vi "MainIdent RT.vi"() -> ()   [LabVIEW 2019]
doc: "The myRIO Project template acquires acceleration data from the onboard accelerometer and displays the changes of acceleration values in a waveform chart."
uses:
  <vilib>/myRIO/Common/Instrument Driver Framework/myRIO v1.0/Encoder/typedefs/Encoder Signal Mode.ctl
  <vilib>/Platform/TimedLoop/XDataNode/timing_clust.ctl
  <vilib>/Platform/TimedLoop/XDataNode/nitl_modes.ctl
  <vilib>/Platform/TimedLoop/XDataNode/wakeup.ctl
  CD1.ctl
  <vilib>/myRIO/Instrument Drivers/Onboard IO/DIO/typedefs/DIO Reference.ctl
  <vilib>/myRIO/Common/Instrument Driver Framework/Utilities/typedefs/myRIO Generic Hardware Reference.ctl
  <vilib>/myRIO/Common/Instrument Driver Framework/Utilities/typedefs/Hardware Version Enum.ctl
  <vilib>/myRIO/Common/Instrument Driver Framework/Utilities/typedefs/myRIO v1.0 Reference.ctl
  <vilib>/myRIO/Common/Instrument Driver Framework/Utilities/typedefs/Generic FPGA Reference.ctl
  <vilib>/myRIO/Common/Instrument Driver Framework/myRIO v1.0/DIO/typedefs/DIO Channels List.ctl
  <vilib>/myRIO/Common/Instrument Driver Framework/myRIO v1.0/DIO/typedefs/DIO Channels Enum.ctl
  <vilib>/userDefined/High Color/nirio_resource_hc.ctl
  <vilib>/myRIO/Common/Instrument Driver Framework/myRIO v1.0/DIO/vis/myRIO v1.1 Open DIO.vi
  3447d3bf-b8a8-43f1-b6f9-cc57a033e7fd.vi
  468b4709-11a8-4de7-9d16-8f3761c489fc.vi
  a2f579e5-2875-4057-bc92-a0e59aafcda8.vi
  <vilib>/myRIO/Common/Instrument Driver Framework/Utilities/vis/Validate Channels.vi
  <vilib>/myRIO/Common/Instrument Driver Framework/myRIO v1.0/DIO/vis/myRIO v1.0 Reserve DIO.vi
  <vilib>/myRIO/Common/Instrument Driver Framework/myRIO v1.0/UART/vis/myRIO v1.0 Close UART.vi
  <vilib>/myRIO/Common/Instrument Driver Framework/myRIO v1.0/Resource Manager/vis/myRIO v1.0 Reserve Channel List.vi
  <vilib>/myRIO/Common/Instrument Driver Framework/myRIO v1.0/DIO/vis/myRIO v1.0 Build MUX Configuration DIO.vi
  <vilib>/myRIO/Common/Instrument Driver Framework/myRIO v1.0/Resource Manager/vis/myRIO v1.0 Reserve Channel.vi
  <vilib>/myRIO/Common/Instrument Driver Framework/myRIO v1.0/Resource Manager/vis/myRIO v1.0 Unreserve Channel.vi
  <vilib>/myRIO/Common/Instrument Driver Framework/myRIO v1.0/Resource Manager/vis/myRIO v1.0 Create Configuration List.vi
  <vilib>/myRIO/Common/Instrument Driver Framework/myRIO v1.0/Resource Manager/vis/myRIO v1.0 Build Mutex Name.vi
  <vilib>/imath/engines/lvmath2/RunTimeEngine/IndexRead/NIMS V(S).vi
  <instcachedir>/0/NIMS V(S)_0488751826AF41519A22953C041130DC.lvgen/NIMS V(S)_0488751826AF41519A22953C041130DC_000.vi
  <vilib>/imathl/engines/lvmath/Functions/Error Handling/Create Error.vi
  <vilib>/imath/engines/lvmath2/RunTimeEngine/ErrorHandling/NIMS_Create Error From Enums.vi
  <vilib>/imath/engines/lvmath2/RunTimeEngine/RangeToken/NIMS_Range_R3 - Integer.vi
  <instcachedir>/0/NIMS_Range_R3 - Integer_E6E7B420460D4F08A65C42474AF91D7C.lvgen/NIMS_Range_R3 - Integer_E6E7B420460D4F08A65C42474AF91D7C_000.vi
  <vilib>/imath/engines/lvmath2/RunTimeEngine/CommandStatement/MC_CommandStatement_break.vi
  <vilib>/imath/engines/lvmath2/RunTimeEngine/VariableToken/NIMS_VariableToken_CondDefinedDefinedByReplace.vi
  <instcachedir>/0/NIMS_VariableToken_CondDefinedDefinedByReplace_D162CFFC24174562A9FEA619A91E1A56.lvgen/NIMS_VariableToken_CondDefinedDefinedByReplace_D162CFFC24174562A9FEA619A91E1A56_003.vi
  <vilib>/imath/engines/lvmath2/RunTimeEngine/IndexReplace/NIMS V(S)=S.vi
  <instcachedir>/0/NIMS V(S)=S_BD5C8CB81B6E4D99B8C0034EA1BEE55D.lvgen/NIMS V(S)=S_BD5C8CB81B6E4D99B8C0034EA1BEE55D_000.vi
  <vilib>/imath/engines/lvmath2/RunTimeEngine/VariableToken/NIMS_VariableToken_CondDefined.vi
  <instcachedir>/0/NIMS_VariableToken_CondDefined_30C3C94EAC01413DA882E848DEC89944.lvgen/NIMS_VariableToken_CondDefined_30C3C94EAC01413DA882E848DEC89944_004.vi
  <vilib>/imath/engines/lvmath/Functions/Error Handling/MergeErrorsWrapper.vi
  <vilib>/imath/engines/lvmath2/RunTimeEngine/NodeEndStatement/NIMS_NodeEndStatement_Output.vi
  <instcachedir>/0/NIMS_NodeEndStatement_Output_53EC0D466D134D7ABD903AC30B43404B.lvgen/NIMS_NodeEndStatement_Output_53EC0D466D134D7ABD903AC30B43404B_001.vi
  <instcachedir>/0/NIMS_NodeEndStatement_Output_53EC0D466D134D7ABD903AC30B43404B.lvgen/NIMS_NodeEndStatement_Output_53EC0D466D134D7ABD903AC30B43404B_005.vi
  <vilib>/imath/engines/lvmath2/RunTimeEngine/ErrorHandling/NIMS_Finalize Error.vi
  <vilib>/Utility/VariantDataType/GetNumericInfo.vi
  <vilib>/Utility/error.llb/Error Cluster From Error Code.vi
  <vilib>/myRIO/Common/Instrument Driver Framework/myRIO v1.0/myRIO v1.1 Open.vi
  <vilib>/myRIO/Common/Instrument Driver Framework/Utilities/vis/IO Manager.vi
  <vilib>/myRIO/Common/Instrument Driver Framework/Utilities/vis/Configuration Manager.vi
  <vilib>/myRIO/Common/Instrument Driver Framework/myRIO v1.0/Resource Manager/vis/myRIO v1.0 Configure IO.vi
  <vilib>/myRIO/Common/Instrument Driver Framework/myRIO v1.0/myRIO v1.0 Close.vi
  <vilib>/myRIO/Common/Instrument Driver Framework/myRIO v1.0/DIO/vis/myRIO v1.0 Read DIO.vi
  <vilib>/myRIO/Common/Instrument Driver Framework/myRIO v1.0/Encoder/vis/myRIO v1.0 Read Encoder.vi
  <vilib>/myRIO/Common/Instrument Driver Framework/myRIO v1.0/DIO/vis/myRIO v1.0 Write DIO.vi
  <vilib>/myRIO/Common/Instrument Driver Framework/myRIO v1.0/PWM/vis/myRIO v1.0 Write PWM.vi
  <vilib>/myRIO/Common/Instrument Driver Framework/Utilities/vis/FPGA Ref Manager.vi
  <vilib>/myRIO/Common/Instrument Driver Framework/myRIO v1.0/myRIO v1.0 Reset FPGA.vi
  <vilib>/myRIO/Common/Instrument Driver Framework/myRIO v1.0/IRQ/vis/myRIO v1.0 IRQ Info FGV.vi
  <vilib>/myRIO/Common/Instrument Driver Framework/myRIO v1.0/IRQ/vis/myRIO v1.0 Timer IRQ Info FGV.vi
  <vilib>/myRIO/Common/Instrument Driver Framework/myRIO v1.0/IRQ/vis/myRIO v1.0 ISR Agent.vi
  <vilib>/myRIO/Instrument Drivers/Utilities/vis/Reset Index.vi
  <vilib>/myRIO/Common/Instrument Driver Framework/myRIO v1.0/Resource Manager/vis/myRIO v1.0 Block Write Resource Manager.vi
  <vilib>/platform/TimedLoop/XDataNode/XDataNode.xnode
  <vilib>/myRIO/Instrument Drivers/Onboard IO/DIO/vis/myRIO DIO Open.xnode
  <vilib>/Platform/TimedLoop/XDataNode/XDNodeRunTimeDep.lvlib
  <vilib>/myRIO/Instrument Drivers/Onboard IO/Encoder/Encoder.lvlib
  <vilib>/myRIO/Instrument Drivers/Onboard IO/PWM/PWM.lvlib
  <vilib>/myRIO/Instrument Drivers/Onboard IO/DIO/DIO.lvlib
  <vilib>/myRIO/Instrument Drivers/Utilities/Utilities.lvlib
panel:
  out "SetPoint Control 4":dbl
  out "Boolean":bool
  out "SetPoint Control 3":dbl
  out "Pos act":dbl
  out "tt_1":dbl[](array[numeric])
  out "SetPoint Control 2":dbl
  out "Td2":dbl
  out "Ti2":dbl
  out "Kp2":dbl
  out "Td1":dbl
  out "Ti1":dbl
  out "Kp1":dbl
  in  "Wc filtro digital 2":dbl
  in  "Wc filtro digital":dbl
  out "Tiempo de muestreo":dbl
  out "Pulsos 1":i32
  out "Pulsos 2":i32
  out "?":cluster{dbl, dbl}(graph)
  out "?":cluster{dbl, dbl}(graph)
  out "Angulo Motor 1":dbl
  out "Angulo Motor 2":dbl
  out "Velocidad Motor1":dbl caption="rad/s"
  out "Velocidad Motor2":dbl caption="rad/s"
  out "Waveform Chart":dbl(graph)
  in  "error":dbl
  in  "error 2":dbl
  out "Numeric":dbl
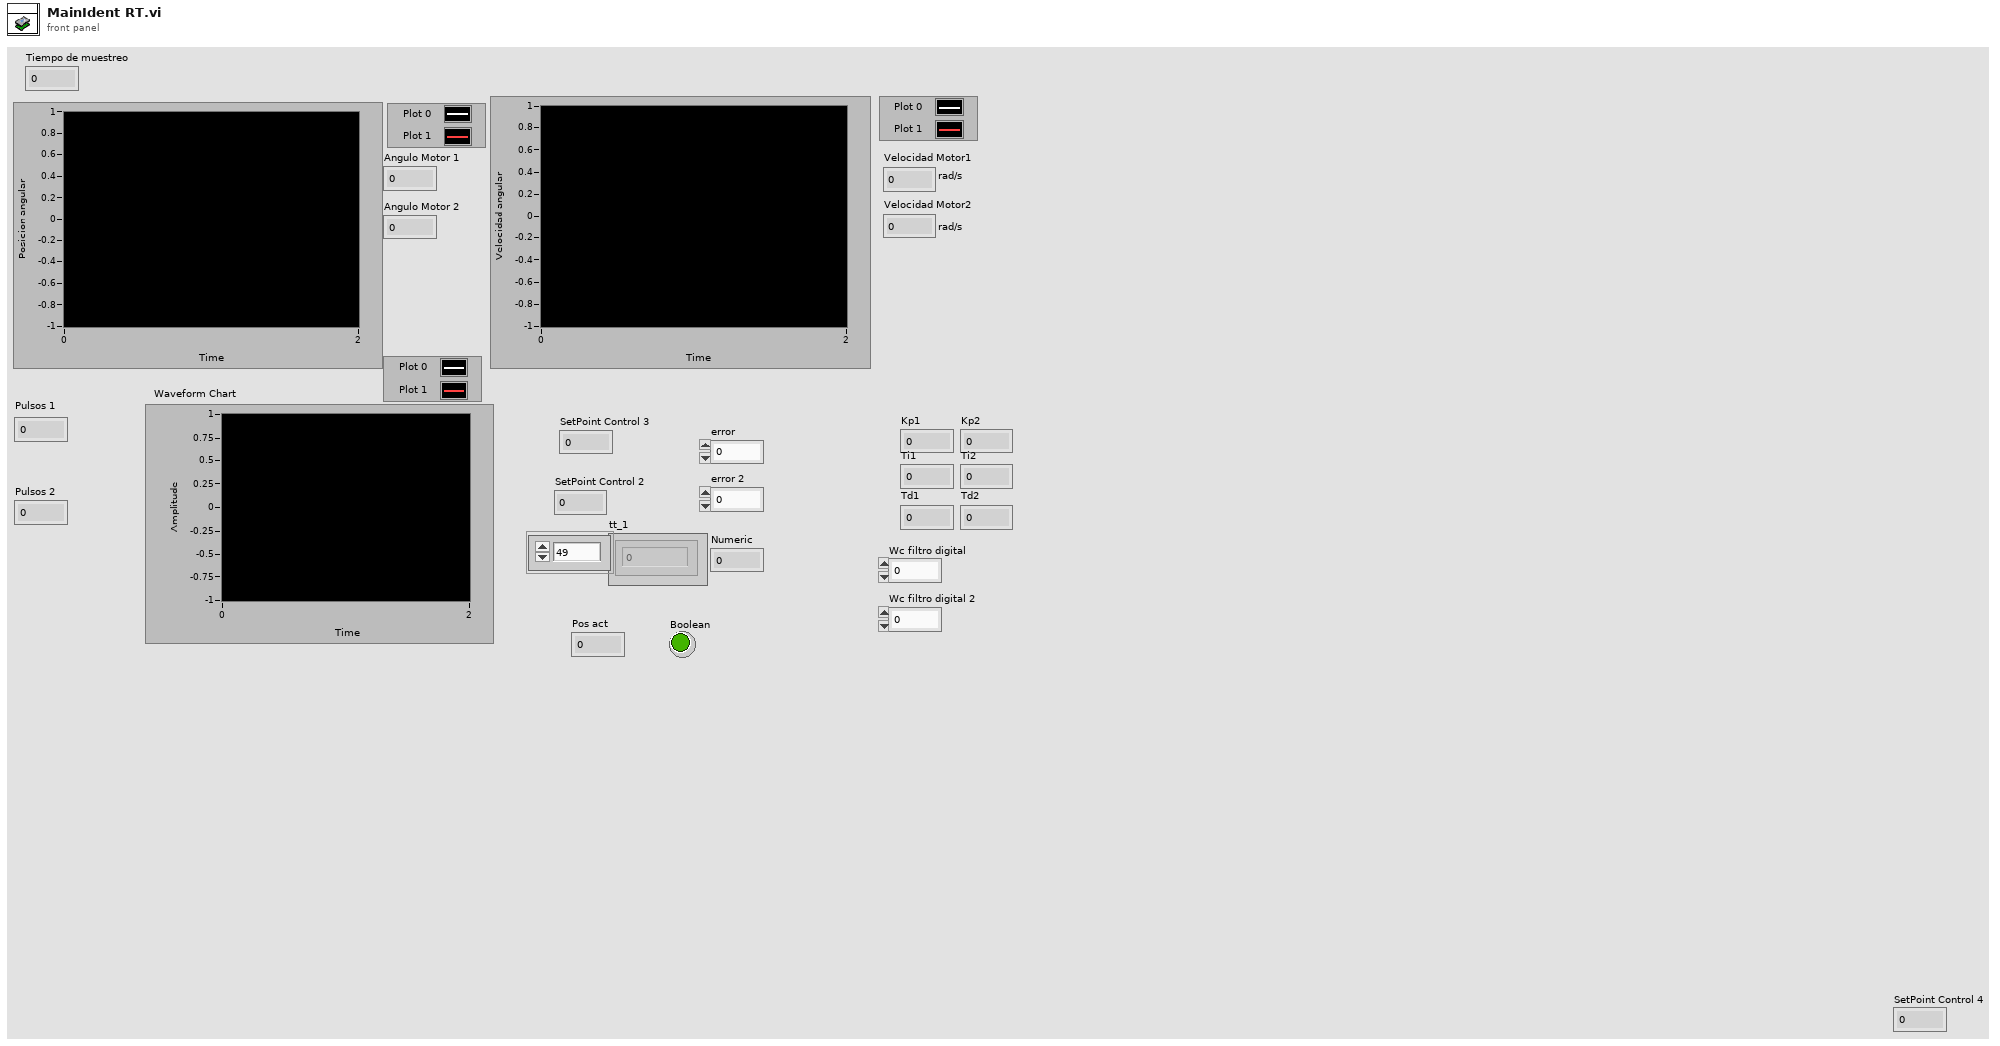
[diagram p1: front panel]
types:
  T1 = typedef "nirio_resource_hc.ctl" = tag
  T2 = typedef "Hardware Version Enum.ctl" = enum16{"Unknown", "myRIO-1900", "myRIO-1950", "roboRIO", "NI ELVIS RIO CM", "ELVIS III"}
  T3 = typedef "XDNodeRunTimeDep.lvlib/timing_clust.ctl" = cluster{"Expected End [f-1]":u64, "Actual End [f-1]":u64, "Finished Late? [f-1]":bool, "Expected End [i-1]":u64, "Actual End [i-1]":u64, "Finished Late? [i-1]":bool, "Expected Start [i]":u64, "Actual Start [i]":u64, "Expected Start [f]":u64, "Actual Start [f]":u64, "Source Name":string, "Structure Name":string, "Period":i64, "Deadline":i64, "Offset":i64, "Start":i64, "Priority":i32, "Timeout":i32, "Mode":T4, "Wakeup Reason":T5, "Error":errorcluster, "Source Type":string, "Secondary Source Type":string, "Global End Time":u64, "Global Start Time":u64, "Frame Duration":u64, "Iteration Duration":u64, "Assigned CPU":i32, "I/O Scan Engine Mode":u32}
  T4 = typedef "XDNodeRunTimeDep.lvlib/nitl_modes.ctl" = enum32{"No Change", "Process missed periods, maintain original phase", "Discard missed periods, maintain original phase", "Process missed periods, ignore original phase", "Discard missed periods, ignore original phase"}
  T5 = typedef "XDNodeRunTimeDep.lvlib/wakeup.ctl" = enum32{"Normal", "Aborted", "Asynchronous wakeup", "Timing source error", "Timed loop error", "Timeout"}
  T6 = cluster{"Double":dbl, "dbl Scaled Value":dbl, "Output":dbl, "seconds since 1Jan1904":timestamp}
  T7 = typedef "Encoder Signal Mode.ctl" = enum16{"Quadrature phase signal", "Step and direction signal"}
  T8 = typedef "PWM.lvlib/PWM Reference.ctl" = cluster{"myRIO Reference":T9, "PWM Channels Enum":T12, "PWM Configuration":T13}
  T9 = typedef "myRIO Generic Hardware Reference.ctl" = cluster{"myRIO Model":T2, "myRIO Hardware Reference":T10}
  T10 = typedef "myRIO v1.0 Reference.ctl" = cluster{"Generic FPGA Reference":T11, "Allow multiple opens":bool}
  T11 = typedef "Generic FPGA Reference.ctl" = refnum<k20>
  T12 = typedef "PWM Channels Enum.ctl" = enum16{"Not Connected", "C/PWM0", "C/PWM1", "A/PWM0", "A/PWM1", "A/PWM2", "A/PWM3", "A/PWM4", "A/PWM5", "A/PWM6", "A/PWM7", "A/PWM8", "A/PWM9", "A/PWM10", "A/PWM11", "A/PWM12", "A/PWM13", "A/PWM14", "A/PWM15", "A/PWM16", "A/PWM17", "A/PWM18", "A/PWM19", "B/PWM0", "B/PWM1", "B/PWM2", "B/PWM3", "B/PWM4", "B/PWM5", "B/PWM6", "B/PWM7", "B/PWM8", "B/PWM9", "B/PWM10", "B/PWM11", "B/PWM12", "B/PWM13", "B/PWM14", "B/PWM15", "B/PWM16", "B/PWM17", "B/PWM18", "B/PWM19", "PWM/PWM0", "PWM/PWM1", "PWM/PWM2", "PWM/PWM3", "PWM/PWM4", "PWM/PWM5", "PWM/PWM6", "PWM/PWM7", "PWM/PWM8", "PWM/PWM9"}
  T13 = typedef "PWM.lvlib/PWM Configuration.ctl" = cluster{"Frequency":dbl, "Duty Cycle":dbl}
  T14 = typedef "DIO.lvlib/DIO Reference.ctl" = cluster{"myRIO Reference":T9, "DIO Channels List":T15}
  T15 = typedef "DIO Channels List.ctl" = T16[]
  T16 = typedef "DIO Channels Enum.ctl" = enum16{"Not Connected", "C/DIO0", "C/DIO1", "C/DIO2", "C/DIO3", "C/DIO4", "C/DIO5", "C/DIO6", "C/DIO7", "A/DIO0", "A/DIO1", "A/DIO2", "A/DIO3", "A/DIO4", "A/DIO5", "A/DIO6", "A/DIO7", "A/DIO8", "A/DIO9", "A/DIO10", "A/DIO11", "A/DIO12", "A/DIO13", "A/DIO14", "A/DIO15", "A/DIO16", "A/DIO17", "A/DIO18", "A/DIO19", "B/DIO0", "B/DIO1", "B/DIO2", "B/DIO3", "B/DIO4", "B/DIO5", "B/DIO6", "B/DIO7", "B/DIO8", "B/DIO9", "B/DIO10", "B/DIO11", "B/DIO12", "B/DIO13", "B/DIO14", "B/DIO15", "B/DIO16", "B/DIO17", "B/DIO18", "B/DIO19", "LED0", "LED1", "LED2", "LED3", "Button0", "DIO/DIO0", "DIO/DIO1", "DIO/DIO2", "DIO/DIO3", "DIO/DIO4", "DIO/DIO5", "DIO/DIO6", "DIO/DIO7", "DIO/DIO8", "DIO/DIO9", "SPI/CS0", "SPI/CS1", "SPI/CS2", "SPI/CS3", "LED RADIO (Green)", "LED RADIO (Red)", "LED COMM (Green)", "LED COMM (Red)", "LED MODE (Green)", "LED MODE (Red)"}
  T17 = typedef "Encoder.lvlib/Encoder Reference.ctl" = cluster{"myRIO Reference":T9, "Encoder Channels Enum":T18}
  T18 = typedef "Encoder Channels Enum.ctl" = enum16{"Not Connected", "C/ENC0", "C/ENC1", "A/ENC", "A/ENC0", "A/ENC1", "A/ENC2", "A/ENC3", "A/ENC4", "A/ENC5", "A/ENC6", "A/ENC7", "A/ENC8", "A/ENC9", "B/ENC", "B/ENC0", "B/ENC1", "B/ENC2", "B/ENC3", "B/ENC4", "B/ENC5", "B/ENC6", "B/ENC7", "B/ENC8", "B/ENC9", "DIO/ENC0", "DIO/ENC1", "DIO/ENC2", "DIO/ENC3", "DIO/ENC4"}
  T19 = typedef "CD1.ctl" = cluster{"D1":dbl[]}
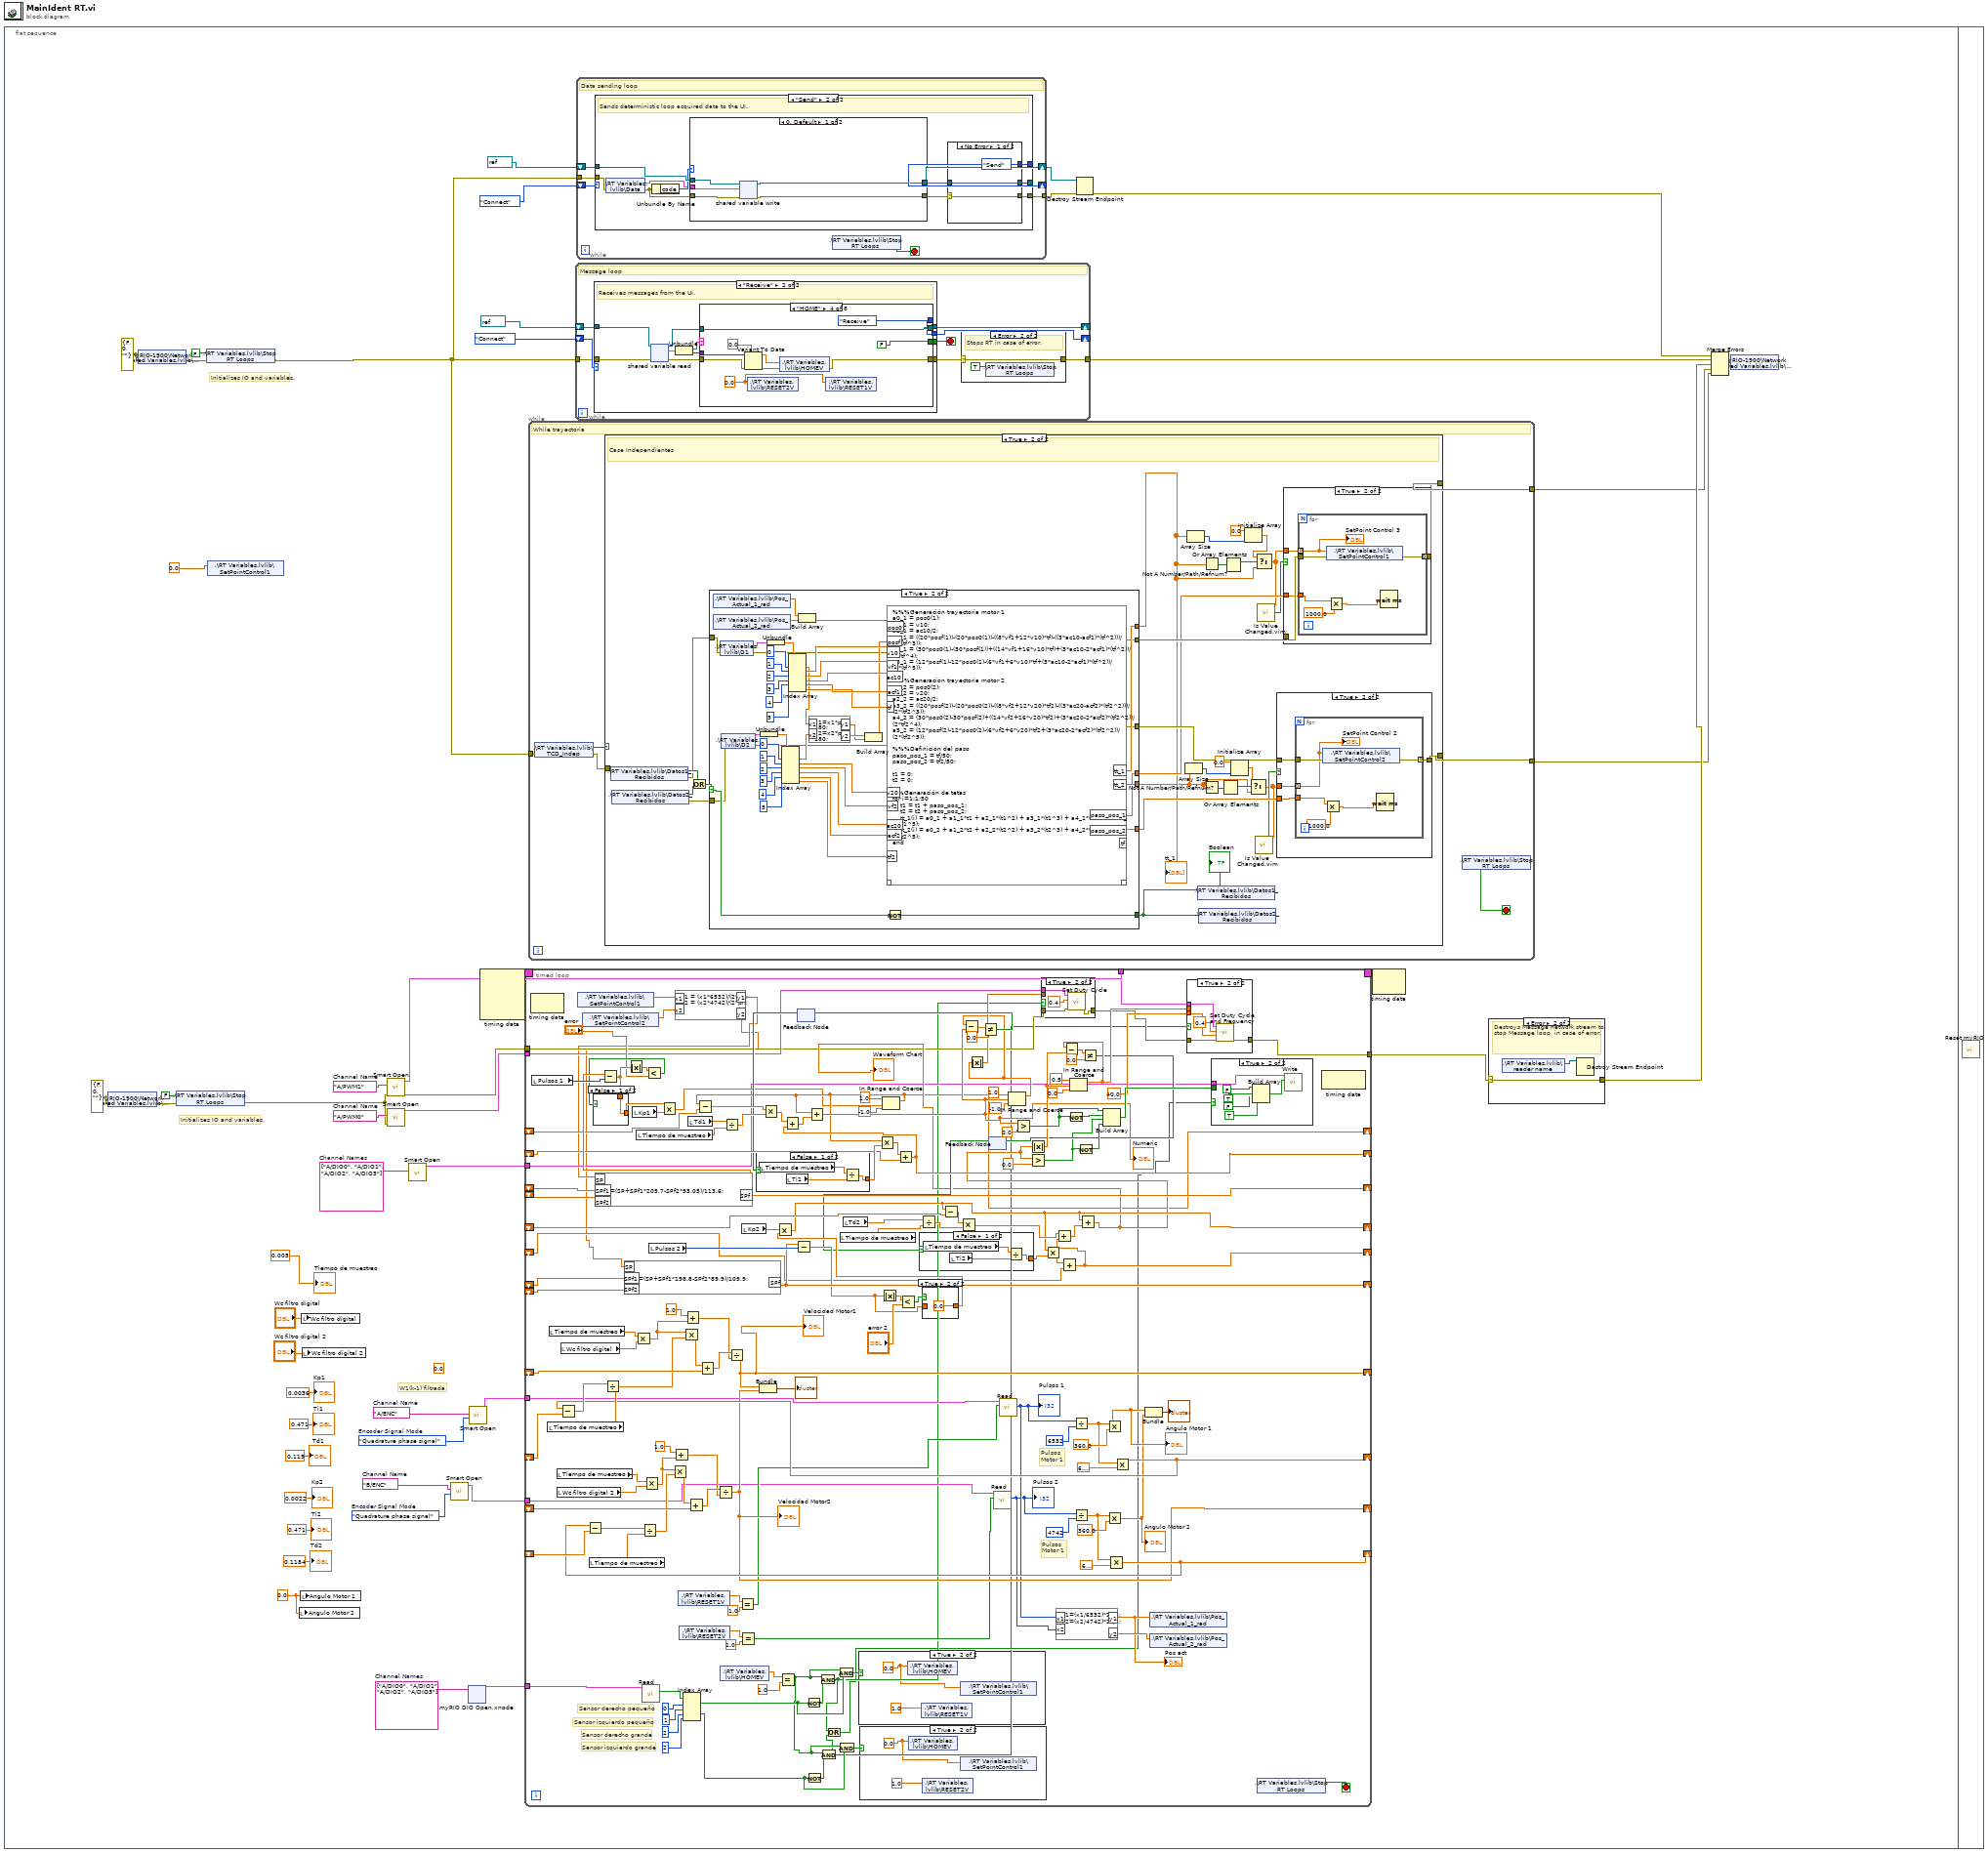
[diagram p0: block diagram]
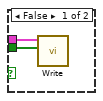
[diagram p4: hidden frame]
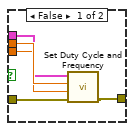
[diagram p5: hidden frame]
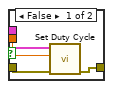
[diagram p6: hidden frame]
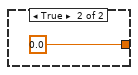
[diagram p7: hidden frame]
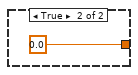
[diagram p8: hidden frame]
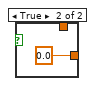
[diagram p10: hidden frame]
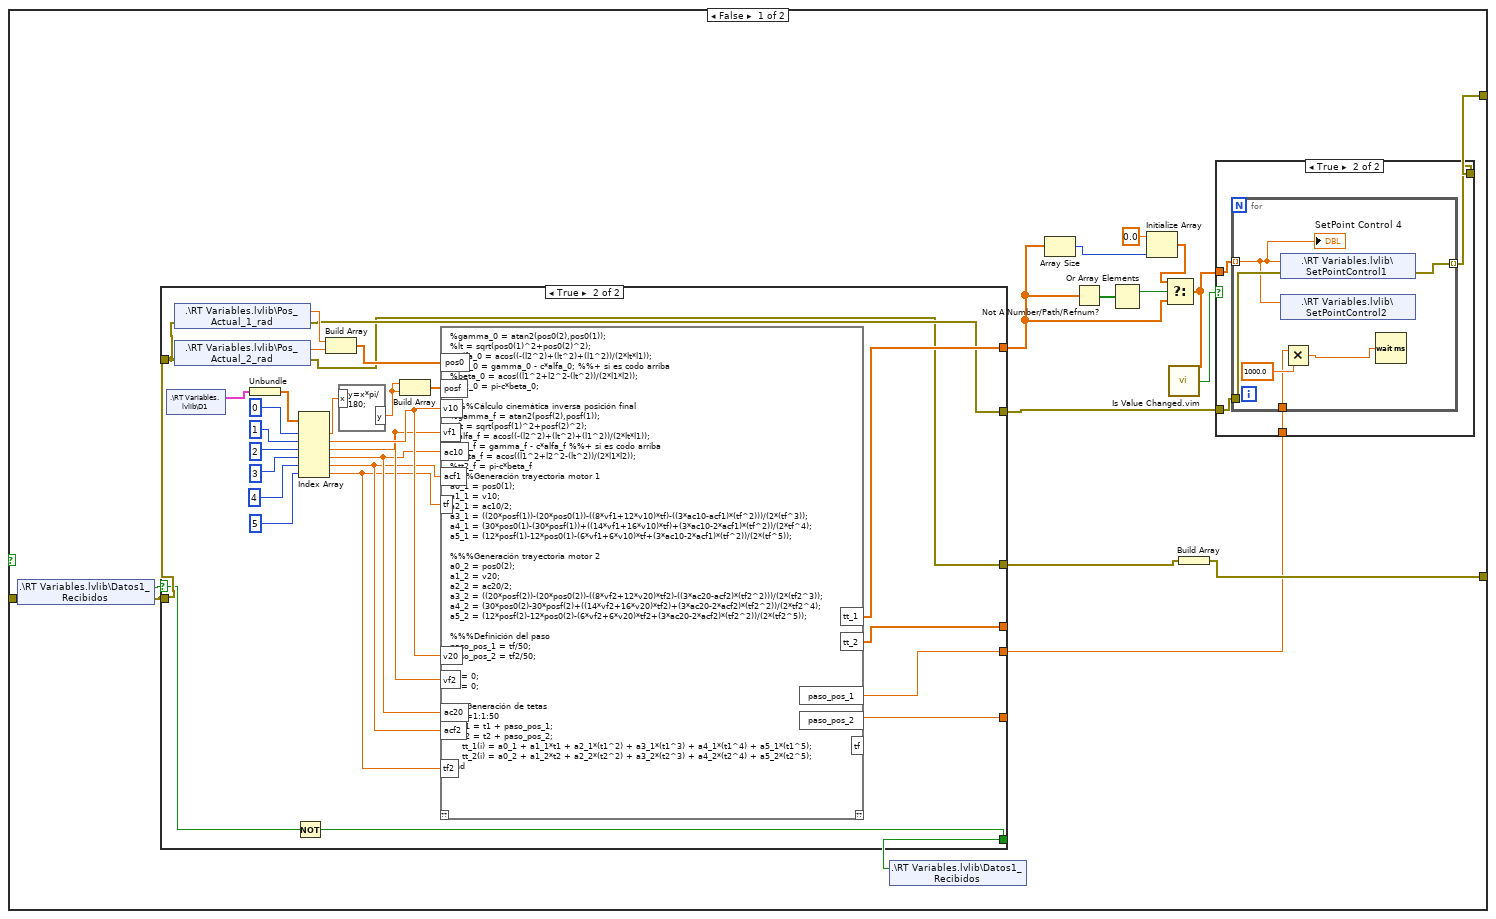
[diagram p11: hidden frame]
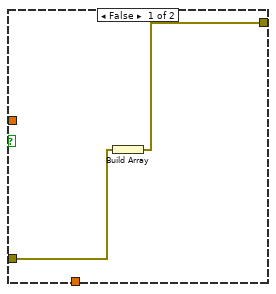
[diagram p12: hidden frame]
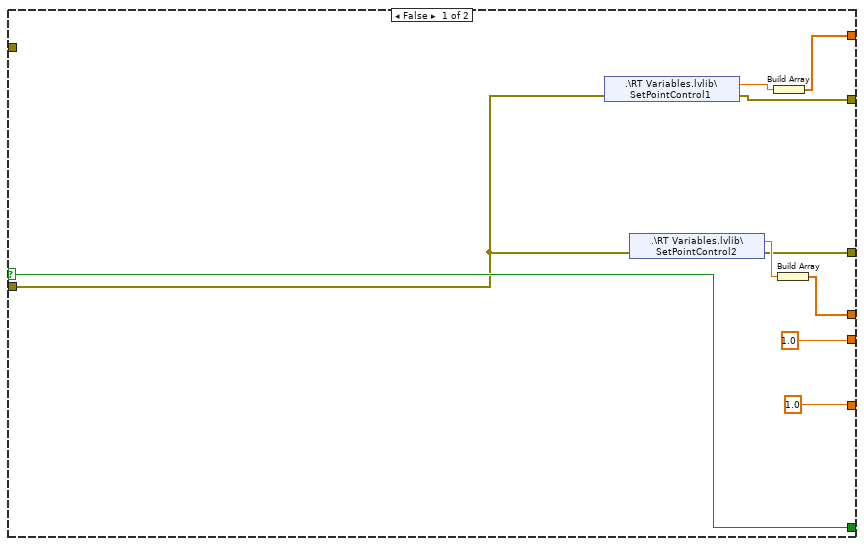
[diagram p13: hidden frame]
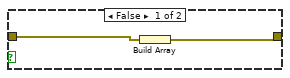
[diagram p14: hidden frame]
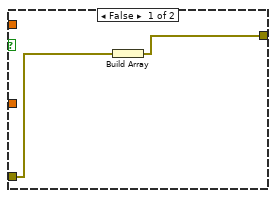
[diagram p15: hidden frame]
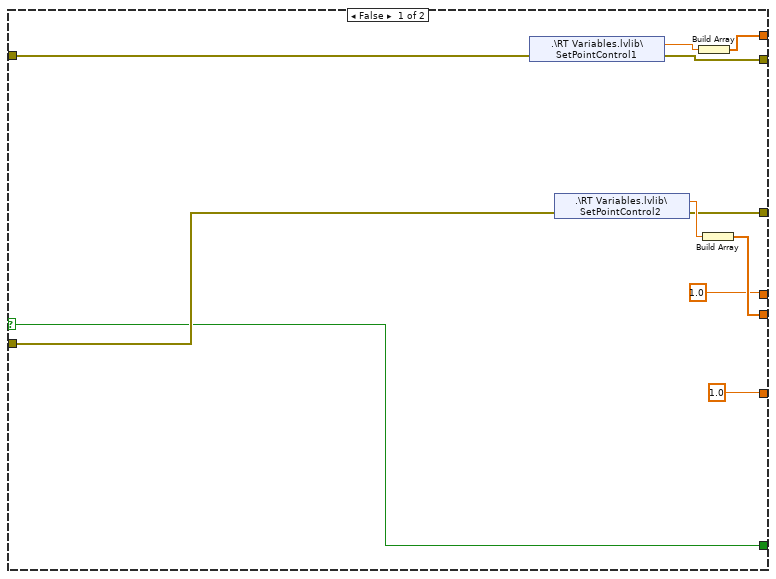
[diagram p16: hidden frame]
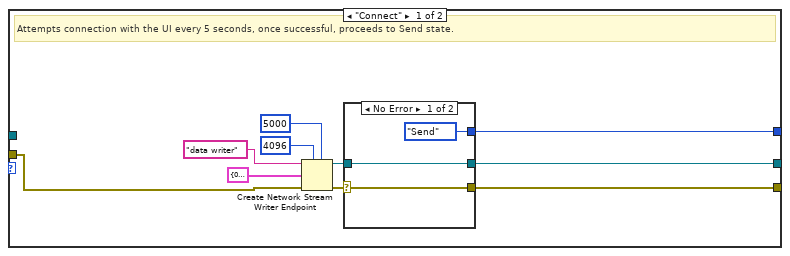
[diagram p18: hidden frame]
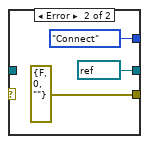
[diagram p19: hidden frame]
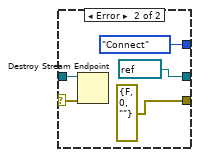
[diagram p20: hidden frame]
diagram:
  n1 = flat-sequence {
    frame #0 {
      w2 = tag[] ["A/DIO0", "A/DIO1", "A/DIO2", "A/DIO3"]  # Channel Names
      w10 = Encoder_Signal_Mode."Quadrature phase signal"  # Encoder Signal Mode
      w9 = tag "B/ENC"  # Channel Name
      w11 = Encoder_Signal_Mode."Quadrature phase signal"  # Encoder Signal Mode
      w13 = tag "A/ENC"  # Channel Name
      w15 = errorcluster {"status"=FALSE, "code"=0, "source"=""} ("error IO")
      w28 = tag "A/PWM1"  # Channel Name
      (unwired) 0.0
      w29 = 0.0 ("Angulo Motor 1")
      w30 = tag[] ["A/DIO0", "A/DIO1", "A/DIO2", "A/DIO3"]  # Channel Names
      w34 = tag "A/PWM0"  # Channel Name
      w36 = errorcluster {"status"=FALSE, "code"=0, "source"=""} ("error IO")
      # "Initializes IO and variables."
      # "W1(k-1) filtrada"
      # "Initializes IO and variables."
      n2 = shared-variable "myRIO-1900\\Network Shared Variables.lvlib\\error IO"(w15, error in=w15) -> (error out=w16:errorcluster)
      n3 = shared-variable "myRIO-1900\\Network Shared Variables.lvlib\\error IO"(w36, error in=w36) -> (error out=w37:errorcluster)
      n4 = shared-variable ".\\RT Variables.lvlib\\Stop RT Loops"(FALSE ("Stop RT Loops"), error in=w16) -> (error out=w14:errorcluster)
      n5 = shared-variable ".\\RT Variables.lvlib\\Stop RT Loops"(FALSE ("Stop RT Loops"), error in=w37) -> (error out=w4:errorcluster)
      n6 = shared-variable ".\\RT Variables.lvlib\\SetPointControl1"(0.0) -> ()  [unwired: 1 in, 1 out]
      n7 = local write "Angulo Motor 2"(w29) -> ()
      n8 = local write "Angulo Motor 1"(w29) -> ()
      n9 = local write "Wc filtro digital"("Wc filtro digital") -> ()
      n10 = local write "Wc filtro digital 2"("Wc filtro digital 2") -> ()
      n11 = call <vilib>:"Smart Open.vi"("error in (no error)"=w14, "Channel Name"=w28) -> ("error out"=w18:errorcluster, "PWM Ref Out"=w21:T8)  [unwired: 8 in]
      n12 = call <vilib>:"Smart Open.vi"("error in (no error)"=w14, "Channel Name"=w34) -> ("PWM Ref Out"=w20:T8)  [unwired: 8 in, 1 out]
      n13 = call <vilib>:"Smart Open.vi"("Channel Names"=w30) -> ("DIO Ref Out"=w19:T14)  [unwired: 9 in, 1 out]
      n14 = call <vilib>:"Smart Open.vi"("Encoder Signal Mode"=w10, "Channel Name"=w9) -> ("Encoder Ref Out"=w8:T17)  [unwired: 8 in, 1 out]
      n15 = xnode "myRIO DIO Open.xnode"("Channel Names"=w2) -> ("DIO Ref Out"=w1:T14)  [unwired: 2 in, 1 out]
      n16 = call <vilib>:"Smart Open.vi"("Encoder Signal Mode"=w11, "Channel Name"=w13) -> ("Encoder Ref Out"=w12:T17)  [unwired: 8 in, 1 out]
      n17 = node-c288() -> (w49:T3)  [unwired: 4 in]
      n18 = timed-loop {
        timing: w49 -> [_]
        timing-out: [_] -> w48
        shift-right: [w208] -> _
        shift-left: _ -> [w209]
        shift-right: [w185] -> _
        shift-left: _ -> [w210]
        shift-right: [w181] -> _
        shift-left: _ -> [w198]
        shift-right: [w180] -> _
        shift-left: _ -> [w187]
        shift-right: [w127] -> _
        shift-left: _ -> [w128]
        shift-right: [w124] -> _
        shift-left: _ -> [w132]
        shift-right: [w167] -> _
        shift-left: _ -> [w169]
        shift-left: _ -> [w168]
        shift-right: [w162] -> _
        shift-left: _ -> [w165]
        shift-left: _ -> [w164]
        shift-right: [w109] -> _
        shift-left: _ -> [w149]
        shift-right: [w145] -> _
        shift-left: _ -> [w146]
        tunnel: w21 -> [w106]
        tunnel: w20 -> [w105]
        tunnel: w19 -> [w104]
        tunnel: w18 -> [w103]
        tunnel: [w101] -> w7
        tunnel: w12 -> [w91]
        tunnel: w8 -> [w90]
        tunnel: w1 -> [w83]
        stop <- w100 stop-if-true
        # "Sensor izquierdo grande"
        # "Sensor derecho grande"
        # "Sensor izquierdo pequeño"
        # "Sensor derecho pequeño"
        # "Pulsos\nMotor 1"
        # "Pulsos\nMotor 1"
        n19 = node-c288() -> ()  [unwired: 1 in, 1 out]
        n20 = local read "Pulsos 1"() -> (w163:i32)
        n21 = local read "Tiempo de muestreo"() -> (w204:dbl)
        n22 = local read "Tiempo de muestreo"() -> (w201:dbl)
        n23 = local read "Tiempo de muestreo"() -> (w200:dbl)
        n24 = local read "Wc filtro digital 2"() -> (w199:dbl)
        n25 = local read "Wc filtro digital"() -> (w202:dbl)
        n26 = shared-variable ".\\RT Variables.lvlib\\SetPointControl1"() -> (w89:dbl)  [unwired: 1 in, 1 out]
        n27 = shared-variable ".\\RT Variables.lvlib\\SetPointControl2"() -> (w88:dbl)  [unwired: 1 in, 1 out]
        n28 = local read "Tiempo de muestreo"() -> (w203:dbl)
        n29 = local read "Kp1"() -> (w155:dbl)
        n30 = Multiply(x=w201, y=w202) -> (x*y=w188:dbl)
        n31 = local read "Tiempo de muestreo"() -> (w153:dbl)
        n32 = call <vilib>:"Read.vi"("DIO Ref In"=w83) -> ("Values"=w82:bool[])  [unwired: 8 in, 2 out]
        n33 = Multiply(x=w200, y=w199) -> (x*y=w195:dbl)
        n34 = local read "Pulsos 2"() -> (w170:i32)
        n35 = Add(x=1.0, y=w195) -> (x+y=w192:dbl)
        n36 = formula code="y1 = (x1*6532)/(2*pi);\ny2 = (x2*4742)/(2*pi);"("x1"=w89, "x2"=w88) -> ("y1"=w87:dbl, "y2"=w86:dbl)
        n37 = formula code="SPf=(SP+SPf1*205.7-SPf2*93.05)/113.6;"("SPf1"=w165, "SPf2"=w164, "SP"=w87) -> ("SPf"=w162:dbl)
        n38 = Subtract(x=w162, y=w163) -> (x-y=w159:dbl)
        n39 = formula code="SPf=(SP+SPf1*198.8-SPf2*89.9)/109.9;"("SPf1"=w169, "SPf2"=w168, "SP"=w86) -> ("SPf"=w167:dbl)
        n40 = Absolute Value(x=w159) -> (abs(x)=w161:dbl)
        n41 = Less?(x=w161, y="error") -> (x < y?=w160:bool)
        n42 = case shown="False" w160 {
          tunnel: [w260 0.0] -> w154
          tunnel: w159 -> [w260 _]
          frame False {
          }
          frame True {
          }
        }
        n43 = Multiply(x=w154, y=w155) -> (x*y=w108:dbl)
        n44 = shared-variable ".\\RT Variables.lvlib\\RESET1V"() -> (w99:dbl)  [unwired: 1 in, 1 out]
        n45 = shared-variable ".\\RT Variables.lvlib\\RESET2V"() -> (w98:dbl)  [unwired: 1 in, 1 out]
        n46 = Index Array(array=w82, index #1=0, index #2=1, index #3=2, index #4=2) -> (element #1=w74:bool, element #3=w69:bool)  [unwired: 2 out]
        n47 = Add(x=1.0, y=w188) -> (x+y=w189:dbl)
        n48 = local read "Td1"() -> (w152:dbl)
        n49 = shared-variable ".\\RT Variables.lvlib\\HOMEV"() -> (w77:dbl)  [unwired: 1 in, 1 out]
        n50 = Divide(x=w152, y=w153) -> (x/y=w151:dbl)
        n51 = Equal?(x=w99, y=1.0) -> (x = y?=w95:bool)
        n52 = Equal?(x=w98, y=1.0) -> (x = y?=w94:bool)
        n53 = local read "Kp2"() -> (w135:dbl)
        n54 = Equal?(x=w77, y=1.0) -> (x = y?=w70:bool)
        n55 = Subtract(x=w167, y=w170) -> (x-y=w134:dbl)
        n56 = feedback #1() -> (w139:bool)  [unwired: 1 in]
        n57 = case shown="False" w139 {
          tunnel: [w254 0.0] -> w148
          frame False {
            n58 = local read "Tiempo de muestreo"() -> (w255:dbl)
            n59 = local read "Ti1"() -> (w256:dbl)
            n60 = Divide(x=w255, y=w256) -> (x/y=w254:dbl)
          }
          frame True {
          }
        }
        n61 = Not(x=w74) -> (.not. x?=w75:bool)
        n62 = Not(x=w69) -> (.not. x?=w72:bool)
        n63 = And(x=w70, y=w75) -> (x .and. y?=w68:bool)
        n64 = And(x=w70, y=w72) -> (x .and. y?=w66:bool)
        n65 = Or(x=w68, y=w66) -> (x .or. y?=w67:bool)
        n66 = And(x=w70, y=w74) -> (x .and. y?=w73:bool)
        n67 = And(x=w70, y=w69) -> (x .and. y?=w71:bool)
        n68 = local read "Tiempo de muestreo"() -> (w138:dbl)
        n69 = local read "Td2"() -> (w137:dbl)
        n70 = case shown="True" w73 {
          frame False {
          }
          frame True {
            w222 = 0.0
            n71 = shared-variable ".\\RT Variables.lvlib\\HOMEV"(w222) -> ()  [unwired: 1 in, 1 out]
            n72 = shared-variable ".\\RT Variables.lvlib\\RESET1V"(1.0) -> ()  [unwired: 1 in, 1 out]
            n73 = shared-variable ".\\RT Variables.lvlib\\SetPointControl1"(w222) -> ()  [unwired: 1 in, 1 out]
          }
        }
        n74 = case shown="True" w71 {
          frame False {
          }
          frame True {
            w220 = 0.0
            n75 = shared-variable ".\\RT Variables.lvlib\\HOMEV"(w220) -> ()  [unwired: 1 in, 1 out]
            n76 = shared-variable ".\\RT Variables.lvlib\\RESET2V"(1.0) -> ()  [unwired: 1 in, 1 out]
            n77 = shared-variable ".\\RT Variables.lvlib\\SetPointControl1"(w220) -> ()  [unwired: 1 in, 1 out]
          }
        }
        n78 = Absolute Value(x=w134) -> (abs(x)=w157:dbl)
        n79 = In Range and Coerce(upper limit=1.0, x=w108, lower limit=-1.0) -> (coerced(x)=w109:dbl)  [unwired: 1 out]
        n80 = Subtract(x=w109, y=w149) -> (x-y=w150:dbl)
        n81 = Multiply(x=w150, y=w151) -> (x*y=w144:dbl)
        n82 = Multiply(x=w109, y=w148) -> (x*y=w147:dbl)
        n83 = Add(x=w147, y=w146) -> (x+y=w145:dbl)
        n84 = Add(x=w144, y=w145) -> (x+y=w143:dbl)
        n85 = Add(x=w109, y=w143) -> (x+y=w113:dbl)
        "Numeric" <- w113
        n86 = Less?(x=w157, y="error 2") -> (x < y?=w117:bool)
        n87 = Divide(x=w137, y=w138) -> (x/y=w136:dbl)
        n88 = case shown="True" w117 {
          tunnel: [w258 0.0] -> w133
          tunnel: w134 -> [w258 _]
          frame False {
          }
          frame True {
          }
        }
        n89 = Multiply(x=w135, y=w133) -> (x*y=w124:dbl)
        n90 = Subtract(x=w124, y=w132) -> (x-y=w131:dbl)
        n91 = Multiply(x=w131, y=w136) -> (x*y=w126:dbl)
        n92 = feedback #2() -> (w118:bool)  [unwired: 1 in]
        n93 = case shown="False" w118 {
          tunnel: [w250 0.0] -> w130
          frame False {
            n94 = local read "Tiempo de muestreo"() -> (w251:dbl)
            n95 = local read "Ti2"() -> (w252:dbl)
            n96 = Divide(x=w251, y=w252) -> (x/y=w250:dbl)
          }
          frame True {
          }
        }
        n97 = call <vilib>:"Read.vi"("Reset Counter"=w94, "Encoder Ref In"=w90) -> ("Counter Value"=w92:i32)  [unwired: 5 in, 4 out]
        "Pulsos 2" <- w92
        n98 = call <vilib>:"Read.vi"("Reset Counter"=w95, "Encoder Ref In"=w91) -> ("Counter Value"=w93:i32)  [unwired: 5 in, 4 out]
        "Pulsos 1" <- w93
        n99 = In Range and Coerce(upper limit=1.0, x=w113, lower limit=-1.0) -> (coerced(x)=w114:dbl)  [unwired: 1 out]
        n100 = Subtract(x=w114, y=w113) -> (x-y=w142:dbl)
        n101 = Absolute Value(x=w114) -> (abs(x)=w115:dbl)
        n102 = Not Equal?(x=w142, y=0.0) -> (x != y?=w140:bool)
        n103 = feedback-in #1(w140) -> ()
        n104 = Greater?(x=w113, y=0.0) -> (0:w166:bool)
        n105 = case shown="True" w68 {
          tunnel: w115 -> [w245 _]
          tunnel: w105 -> [w244 w249]
          tunnel: w103 -> [w243 w247]
          tunnel: [w242 w246] -> w102
          frame False {
            n106 = call <vilib>:"Set Duty Cycle.vi"("error in (no error)"=w243, "Duty Cycle"=w245, "PWM Ref In"=w244) -> ("error out"=w242:errorcluster)  [unwired: 6 in, 1 out]
          }
          frame True {
            n107 = call <vilib>:"Set Duty Cycle.vi"("error in (no error)"=w247, "Duty Cycle"=0.4, "PWM Ref In"=w249) -> ("error out"=w246:errorcluster)  [unwired: 6 in, 1 out]
          }
        }
        n108 = Multiply(x=w124, y=w130) -> (x*y=w129:dbl)
        n109 = formula code="y1=(x1/6532)*2*pi;\ny2=(x2/4742)*2*pi;"("x1"=w93, "x2"=w92) -> ("y1"=w84:dbl, "y2"=w85:dbl)
        "Pos act" <- w84
        n110 = Add(x=w129, y=w128) -> (x+y=w127:dbl)
        n111 = Add(x=w126, y=w127) -> (x+y=w125:dbl)
        n112 = Not(x=w166) -> (.not. x?=w178:bool)
        n113 = Divide(x=w93, y=6532) -> (x/y=w214:dbl)
        n114 = Divide(x=w92, y=4742) -> (x/y=w212:dbl)
        n115 = Add(x=w124, y=w125) -> (x+y=w112:dbl)
        "Waveform Chart" <- w112
        n116 = Absolute Value(x=w112) -> (abs(x)=w123:dbl)
        n117 = Greater?(x=w112, y=0.0) -> (0:w116:bool)
        n118 = In Range and Coerce(upper limit=0.5, x=w123, lower limit=0.0) -> (coerced(x)=w122:dbl)  [unwired: 1 out]
        n119 = Subtract(x=w122, y=w123) -> (x-y=w121:dbl)
        n120 = Not(x=w116) -> (.not. x?=w176:bool)
        n121 = Not Equal?(x=w121, y=0.0) -> (x != y?=w119:bool)
        n122 = feedback-in #2(w119) -> ()
        n123 = Build Array(w166, w178, w116, w176) -> (w182:bool[])
        n124 = Multiply(x=w214, y=360.0) -> (x*y=w184:dbl)
        "Angulo Motor 1" <- w184
        n125 = Multiply(x=w212, y=360.0) -> (x*y=w183:dbl)
        "Angulo Motor 2" <- w183
        n126 = Multiply(x=w212, y=6.283185307179586) -> (x*y=w208:dbl)
        n127 = Subtract(x=w208, y=w209) -> (x-y=w207:dbl)
        n128 = Divide(x=w207, y=w203) -> (x/y=w197:dbl)
        n129 = Multiply(x=w195, y=w197) -> (x*y=w196:dbl)
        n130 = Add(x=w196, y=w198) -> (x+y=w193:dbl)
        n131 = Divide(x=w193, y=w192) -> (x/y=w181:dbl)
        "Velocidad Motor2" <- w181
        n132 = Multiply(x=w214, y=6.283185307179586) -> (x*y=w185:dbl)
        n133 = Subtract(x=w185, y=w210) -> (x-y=w206:dbl)
        n134 = Divide(x=w206, y=w204) -> (x/y=w186:dbl)
        n135 = Multiply(x=w188, y=w186) -> (x*y=w191:dbl)
        n136 = Add(x=w191, y=w187) -> (x+y=w190:dbl)
        n137 = Divide(x=w190, y=w189) -> (x/y=w180:dbl)
        "Velocidad Motor1" <- w180
        n138 = Bundle(w180, w181) -> (→"?":cluster{dbl, dbl})  [unwired: 1 in]
        n139 = Bundle(w184, w183) -> (→"?":cluster{dbl, dbl})  [unwired: 1 in]
        n140 = shared-variable ".\\RT Variables.lvlib\\Pos_Actual_1_rad"(w84) -> ()  [unwired: 1 in, 1 out]
        n141 = shared-variable ".\\RT Variables.lvlib\\Pos_Actual_2_rad"(w85) -> ()  [unwired: 1 in, 1 out]
        n142 = case shown="True" w66 {
          tunnel: w122 -> [w236 _]
          tunnel: 40.0 -> [w235 w238]
          tunnel: w106 -> [w234 w239]
          tunnel: w102 -> [w233 w240]
          tunnel: [w232 w241] -> w101
          frame False {
            n143 = call <vilib>:"Set Duty Cycle and Frequency.vi"("error in (no error)"=w233, "Frequency [Hz]"=w235, "Duty Cycle"=w236, "PWM Ref In"=w234) -> ("error out"=w232:errorcluster)  [unwired: 5 in, 1 out]
          }
          frame True {
            n144 = call <vilib>:"Set Duty Cycle and Frequency.vi"("error in (no error)"=w240, "Frequency [Hz]"=w238, "Duty Cycle"=0.4, "PWM Ref In"=w239) -> ("error out"=w241:errorcluster)  [unwired: 5 in, 1 out]
          }
        }
        n145 = case shown="True" w67 {
          tunnel: w182 -> [w225 _]
          tunnel: w104 -> [w224 w231]
          frame False {
            n146 = call <vilib>:"Write.vi"("Values"=w225, "DIO Ref In"=w224) -> ()  [unwired: 7 in, 2 out]
          }
          frame True {
            n147 = Build Array(FALSE, TRUE, FALSE, TRUE) -> (w226:bool[])
            n148 = call <vilib>:"Write.vi"("Values"=w226, "DIO Ref In"=w231) -> ()  [unwired: 7 in, 2 out]
          }
        }
        n149 = shared-variable ".\\RT Variables.lvlib\\Stop RT Loops"() -> (w100:bool)  [unwired: 1 in, 1 out]
        n150 = node-c288() -> ()  [unwired: 1 in, 1 out]
      }
      n151 = while {
        tunnel: [w267] -> w6
        tunnel: [w266] -> w5
        tunnel: w4 -> [w268]
        stop <- w271 stop-if-true
        # "While trayectoria"
        n152 = shared-variable ".\\RT Variables.lvlib\\TCD_Indep"(error in=w268) -> (w270:bool, error out=w269:errorcluster)
        n153 = case shown="True" w270 {
          tunnel: w269 -> [w286 _]
          tunnel: [w273 w1042] -> w267
          tunnel: [w283 w1045] -> w266
          frame False {
            n154 = shared-variable ".\\RT Variables.lvlib\\Datos1_Recibidos"(error in=w286) -> (w288:bool, error out=w285:errorcluster)
            n155 = case shown="True" w288 {
              selector: w288 -> [w310 w321]
              tunnel: [w310 w320] -> w287
              tunnel: [w307 w317] -> w275
              tunnel: [w306 w316] -> _
              tunnel: [1.0 w315] -> w272
              tunnel: [1.0 w314] -> _
              tunnel: w285 -> [_ w311]
              tunnel: w285 -> [w303 _]
              tunnel: [w302 w313] -> w274
              tunnel: [w301 w312] -> w284
              frame False {
                n156 = shared-variable ".\\RT Variables.lvlib\\SetPointControl1"(error in=w303) -> (w308:dbl, error out=w302:errorcluster)
                n157 = shared-variable ".\\RT Variables.lvlib\\SetPointControl2"(error in=w303) -> (w309:dbl, error out=w301:errorcluster)
                n158 = Build Array(w308) -> (w307:dbl[])
                n159 = Build Array(w309) -> (w306:dbl[])
              }
              frame True {
                n160 = shared-variable ".\\RT Variables.lvlib\\D1"() -> (w334:T19)  [unwired: 1 in, 1 out]
                n161 = shared-variable ".\\RT Variables.lvlib\\Pos_Actual_1_rad"(error in=w311) -> (w338:dbl, error out=w313:errorcluster)
                n162 = shared-variable ".\\RT Variables.lvlib\\Pos_Actual_2_rad"(error in=w311) -> (w337:dbl, error out=w312:errorcluster)
                n163 = Unbundle(w334) -> ("D1"=w335:dbl[])
                n164 = Not(x=w321) -> (.not. x?=w320:bool)
                n165 = Index Array(array=w335, index #1=0, index #2=1, index #3=2, index #4=3, index #5=4, index #6=5) -> (element #1=w318:dbl, element #2=w327:dbl, element #3=w325:dbl, element #4=w324:dbl, element #5=w323:dbl, element #6=w322:dbl)
                n166 = Build Array(w338, w337) -> (w336:dbl[])
                n167 = formula code="y=x*pi/180;"("x"=w318) -> ("y"=w319:dbl)
                n168 = Build Array(w319, w319) -> (w326:dbl[])
                n169 = mathscript code="%gamma_0 = atan2(pos0(2),pos0(1));\n%lt = sqrt(pos0(1)^2+pos0(2)^2);\n%alfa_0 = acos((-(l2^2)+(lt^2)+(l1^2))/(2*lt*l1));\n%tt1_0 = gamma_0 - c*alfa_0; %%+ si es codo arriba\n%beta_0 = acos((l1^2+l2^2-(lt^2))/(2*l1*l2));\n%tt2_0 = pi-c*beta_0;\n\n%%%Cálculo cinemática inversa posición final\n%gamma_f = atan2(posf(2),posf(1));\n%lt = sqrt(posf(1)^2+posf(2)^2);\n%alfa_f = acos((-(l2^2)+(lt^2)+(l1^2))/(2*lt*l1));\n%tt1_f = gamma_f - c*alfa_f %%+ si es codo arriba\n%beta_f = acos((l1^2+l2^2-(lt^2))/(2*l1*l2));\n%tt2_f = pi-c*beta_f\n%%%Generación trayectoria motor 1\na0_1 = pos0(1);\na1_1 = v10;\na2_1 = ac10/2;\na3_1 = ((20*posf(1))-(20*pos0(1))-((8*vf1+12*v10)*tf)-((3*ac10-acf1)*(tf^2)))/(2*(tf^3));\na4_1 = (30*pos0(1)-(30*posf(1))+((14*vf1+16*v10)*tf)+(3*ac10-2*acf1)*(tf^2))/(2*tf^4);\na5_1 = (12*posf(1)-12*pos0(1)-(6*vf1+6*v10)*tf+(3*ac10-2*acf1)*(tf^2))/(2*(tf^5));\n\n%%%Generación trayectoria motor 2\na0_2 = pos0(2);\na1_2 = v20;\na2_2 = ac20/2;\na3_2 = ((20*posf(2))-(20*pos0(2))-((8*vf2+12*v20)*tf2)-((3*ac20-acf2)*(tf2^2)))/(2*(tf2^3));\na4_2 = (30*pos0(2)-30*posf(2)+((14*vf2+16*v20)*tf2)+(3*ac20-2*acf2)*(tf2^2))/(2*tf2^4);\na5_2 = (12*posf(2)-12*pos0(2)-(6*vf2+6*v20)*tf2+(3*ac20-2*acf2)*(tf2^2))/(2*(tf2^5));\n\n%%%Definición del paso\npaso_pos_1 = tf/50;\npaso_pos_2 = tf2/50;\n\nt1 = 0;\nt2 = 0;\n\n%%Generación de tetas\nfor i=1:1:50\n    t1 = t1 + paso_pos_1;\n    t2 = t2 + paso_pos_2;\n    tt_1(i) = a0_1 + a1_1*t1 + a2_1*(t1^2) + a3_1*(t1^3) + a4_1*(t1^4) + a5_1*(t1^5);\n    tt_2(i) = a0_2 + a1_2*t2 + a2_2*(t2^2) + a3_2*(t2^3) + a4_2*(t2^4) + a5_2*(t2^5);\nend"("pos0"=w336, "posf"=w326, "tf"=w322, "v10"=w327, "vf1"=w325, "ac10"=w324, "acf1"=w323, "tf2"=w322, "v20"=w327, "ac20"=w324, "vf2"=w325, "acf2"=w323) -> ("tt_1"=w317:dbl[], "tt_2"=w316:dbl[], "paso_pos_1"=w315:dbl, "paso_pos_2"=w314:dbl)  [unwired: 1 in, 2 out]
              }
            }
            n170 = shared-variable ".\\RT Variables.lvlib\\Datos1_Recibidos"(w287) -> ()  [unwired: 1 in, 1 out]
            n171 = Array Size(array=w275) -> (size(s)=w280:i32)
            n172 = Not A Number/Path/Refnum?(number/path/refnum=w275) -> (NaN/Path/Refnum?=w282:bool[])
            n173 = Or Array Elements(Boolean array=w282) -> (logical OR=w281:bool)
            n174 = Initialize Array(0.0, w280) -> (w278:dbl[])
            n175 = Select(t=w278, s=w281, f=w275) -> (s? t:f=w276:dbl[])
            n176 = call "Is Value Changed.vim"("value"=w276) -> ("changed or first call?"=w277:bool)
            n177 = Build Array(w284) -> (w283:errorcluster[])
            n178 = case shown="True" w277 {
              tunnel: w276 -> [_ w294]
              tunnel: w274 -> [w289 w293]
              tunnel: [w290 w292] -> w273
              tunnel: w272 -> [_ w291]
              frame False {
                n179 = Build Array(w289) -> (w290:errorcluster[])
              }
              frame True {
                n180 = for {
                  tunnel: w294 -> [w296] mode=indexing
                  tunnel: w293 -> [w298]
                  tunnel: [w297] -> w292 mode=indexing
                  tunnel: w291 -> [w295]
                  n181 = shared-variable ".\\RT Variables.lvlib\\SetPointControl1"(w296, error in=w298) -> (error out=w297:errorcluster)
                  n182 = shared-variable ".\\RT Variables.lvlib\\SetPointControl2"(w296) -> ()  [unwired: 1 in, 1 out]
                  n183 = Multiply(x=w295, y=1000.0) -> (x*y=w299:dbl)
                  n184 = Wait (ms)(milliseconds to wait=w299) -> ()  [unwired: 1 out]
                  "SetPoint Control 4" <- w296
                }
              }
            }
          }
          frame True {
            # "Case Independientes"
            n185 = shared-variable ".\\RT Variables.lvlib\\Datos1_Recibidos"() -> (w1052:bool, error out=w1049:errorcluster)  [unwired: 1 in]
            n186 = shared-variable ".\\RT Variables.lvlib\\Datos2_Recibidos"() -> (w1051:bool, error out=w1048:errorcluster)  [unwired: 1 in]
            n187 = Or(x=w1052, y=w1051) -> (x .or. y?=w1050:bool)
            n188 = case shown="True" w1050 {
              selector: w1050 -> [w1077 w1099]
              tunnel: [w1086 w1098] -> w1035
              tunnel: [w1084 w1097] -> w1028
              tunnel: [1.0 w1096] -> w1043
              tunnel: [1.0 w1095] -> w1047
              tunnel: w1049 -> [w1081 w1091]
              tunnel: w1048 -> [w1080 w1092]
              tunnel: [w1079 w1094] -> w1044
              tunnel: [w1078 w1093] -> w1046
              tunnel: [w1077 w1088] -> w1041
              frame False {
                n189 = shared-variable ".\\RT Variables.lvlib\\SetPointControl1"(error in=w1081) -> (w1087:dbl, error out=w1079:errorcluster)
                n190 = shared-variable ".\\RT Variables.lvlib\\SetPointControl2"(error in=w1080) -> (w1085:dbl, error out=w1078:errorcluster)
                n191 = Build Array(w1087) -> (w1086:dbl[])
                n192 = Build Array(w1085) -> (w1084:dbl[])
              }
              frame True {
                n193 = shared-variable ".\\RT Variables.lvlib\\Pos_Actual_1_rad"() -> (w1115:dbl)  [unwired: 1 in, 1 out]
                n194 = shared-variable ".\\RT Variables.lvlib\\Pos_Actual_2_rad"() -> (w1114:dbl)  [unwired: 1 in, 1 out]
                n195 = shared-variable ".\\RT Variables.lvlib\\D1"(error in=w1091) -> (w1131:T19, error out=w1094:errorcluster)
                n196 = shared-variable ".\\RT Variables.lvlib\\D2"(error in=w1092) -> (w1123:T19, error out=w1093:errorcluster)
                n197 = Unbundle(w1123) -> ("D1"=w1122:dbl[])
                n198 = Unbundle(w1131) -> ("D1"=w1130:dbl[])
                n199 = Index Array(array=w1122, index #1=0, index #2=1, index #3=2, index #4=3, index #5=4, index #6=5) -> (element #1=w1102:dbl, element #2=w1107:dbl, element #3=w1106:dbl, element #4=w1105:dbl, element #5=w1104:dbl, element #6=w1103:dbl)
                n200 = Index Array(array=w1130, index #1=0, index #2=1, index #3=2, index #4=3, index #5=4, index #6=5) -> (element #1=w1101:dbl, element #2=w1112:dbl, element #3=w1111:dbl, element #4=w1110:dbl, element #5=w1109:dbl, element #6=w1108:dbl)
                n201 = Build Array(w1115, w1114) -> (w1113:dbl[])
                n202 = formula code="y1=x1*pi/180;\ny2=x2*pi/180;"("x1"=w1101, "x2"=w1102) -> ("y1"=w1090:dbl, "y2"=w1089:dbl)
                n203 = Build Array(w1090, w1089) -> (w1100:dbl[])
                n204 = Not(x=w1099) -> (.not. x?=w1088:bool)
                n205 = mathscript code="%%%Generación trayectoria motor 1\na0_1 = pos0(1);\na1_1 = v10;\na2_1 = ac10/2;\na3_1 = ((20*posf(1))-(20*pos0(1))-((8*vf1+12*v10)*tf)-((3*ac10-acf1)*(tf^2)))/(2*(tf^3));\na4_1 = (30*pos0(1)-(30*posf(1))+((14*vf1+16*v10)*tf)+(3*ac10-2*acf1)*(tf^2))/(2*tf^4);\na5_1 = (12*posf(1)-12*pos0(1)-(6*vf1+6*v10)*tf+(3*ac10-2*acf1)*(tf^2))/(2*(tf^5));\n\n%%%Generación trayectoria motor 2\na0_2 = pos0(2);\na1_2 = v20;\na2_2 = ac20/2;\na3_2 = ((20*posf(2))-(20*pos0(2))-((8*vf2+12*v20)*tf2)-((3*ac20-acf2)*(tf2^2)))/(2*(tf2^3));\na4_2 = (30*pos0(2)-30*posf(2)+((14*vf2+16*v20)*tf2)+(3*ac20-2*acf2)*(tf2^2))/(2*tf2^4);\na5_2 = (12*posf(2)-12*pos0(2)-(6*vf2+6*v20)*tf2+(3*ac20-2*acf2)*(tf2^2))/(2*(tf2^5));\n\n%%%Definición del paso\npaso_pos_1 = tf/50;\npaso_pos_2 = tf2/50;\n\nt1 = 0;\nt2 = 0;\n\n%%Generación de tetas\nfor i=1:1:50\n    t1 = t1 + paso_pos_1;\n    t2 = t2 + paso_pos_2;\n    tt_1(i) = a0_1 + a1_1*t1 + a2_1*(t1^2) + a3_1*(t1^3) + a4_1*(t1^4) + a5_1*(t1^5);\n    tt_2(i) = a0_2 + a1_2*t2 + a2_2*(t2^2) + a3_2*(t2^3) + a4_2*(t2^4) + a5_2*(t2^5);\nend"("pos0"=w1113, "posf"=w1100, "tf"=w1108, "v10"=w1112, "vf1"=w1111, "ac10"=w1110, "acf1"=w1109, "tf2"=w1103, "v20"=w1107, "ac20"=w1105, "vf2"=w1106, "acf2"=w1104) -> ("tt_1"=w1098:dbl[], "tt_2"=w1097:dbl[], "paso_pos_1"=w1096:dbl, "paso_pos_2"=w1095:dbl)  [unwired: 1 in, 2 out]
              }
            }
            "tt_1" <- w1035
            "Boolean" <- w1041
            n206 = Array Size(array=w1028) -> (size(s)=w1031:i32)
            n207 = Array Size(array=w1035) -> (size(s)=w1038:i32)
            n208 = shared-variable ".\\RT Variables.lvlib\\Datos1_Recibidos"(w1041) -> ()  [unwired: 1 in, 1 out]
            n209 = shared-variable ".\\RT Variables.lvlib\\Datos2_Recibidos"(w1041) -> ()  [unwired: 1 in, 1 out]
            n210 = Not A Number/Path/Refnum?(number/path/refnum=w1035) -> (NaN/Path/Refnum?=w1040:bool[])
            n211 = Not A Number/Path/Refnum?(number/path/refnum=w1028) -> (NaN/Path/Refnum?=w1027:bool[])
            n212 = Or Array Elements(Boolean array=w1027) -> (logical OR=w1032:bool)
            n213 = Or Array Elements(Boolean array=w1040) -> (logical OR=w1039:bool)
            n214 = Initialize Array(0.0, w1031) -> (w1029:dbl[])
            n215 = Initialize Array(0.0, w1038) -> (w1036:dbl[])
            n216 = Select(t=w1029, s=w1032, f=w1028) -> (s? t:f=w1025:dbl[])
            n217 = Select(t=w1036, s=w1039, f=w1035) -> (s? t:f=w1033:dbl[])
            n218 = call "Is Value Changed.vim"("value"=w1025) -> ("changed or first call?"=w1026:bool)
            n219 = call "Is Value Changed.vim"("value"=w1033) -> ("changed or first call?"=w1034:bool)
            n220 = case shown="True" w1026 {
              tunnel: w1047 -> [_ w1058]
              tunnel: w1046 -> [w1054 w1057]
              tunnel: [w1053 w1056] -> w1045
              tunnel: w1025 -> [_ w1055]
              frame False {
                n221 = Build Array(w1054) -> (w1053:errorcluster[])
              }
              frame True {
                n222 = for {
                  tunnel: w1058 -> [w1062]
                  tunnel: w1057 -> [w1061]
                  tunnel: [w1060] -> w1056 mode=indexing
                  tunnel: w1055 -> [w1059] mode=indexing
                  n223 = shared-variable ".\\RT Variables.lvlib\\SetPointControl2"(w1059, error in=w1061) -> (error out=w1060:errorcluster)
                  n224 = Multiply(x=w1062, y=1000.0) -> (x*y=w1063:dbl)
                  n225 = Wait (ms)(milliseconds to wait=w1063) -> ()  [unwired: 1 out]
                  "SetPoint Control 2" <- w1059
                }
              }
            }
            n226 = case shown="True" w1034 {
              tunnel: w1044 -> [w1066 w1070]
              tunnel: w1043 -> [_ w1069]
              tunnel: [w1065 w1068] -> w1042
              tunnel: w1033 -> [_ w1067]
              frame False {
                n227 = Build Array(w1066) -> (w1065:errorcluster[])
              }
              frame True {
                n228 = for {
                  tunnel: w1069 -> [w1072]
                  tunnel: w1070 -> [w1074]
                  tunnel: [w1073] -> w1068 mode=indexing
                  tunnel: w1067 -> [w1071] mode=indexing
                  n229 = shared-variable ".\\RT Variables.lvlib\\SetPointControl1"(w1071, error in=w1074) -> (error out=w1073:errorcluster)
                  n230 = Multiply(x=w1072, y=1000.0) -> (x*y=w1075:dbl)
                  n231 = Wait (ms)(milliseconds to wait=w1075) -> ()  [unwired: 1 out]
                  "SetPoint Control 3" <- w1071
                }
              }
            }
          }
        }
        n232 = shared-variable ".\\RT Variables.lvlib\\Stop RT Loops"() -> (w271:bool)  [unwired: 1 in, 1 out]
      }
      n233 = while {
        tunnel: [w1870] -> w39
        shift-right: [w1876] -> _
        shift-left: refnum<k21> refnum ("reader name") -> [w1874]
        shift-right: [w1875] -> _
        shift-left: enum16{"Connect", "Receive"}."Connect" ("Message states") -> [w1877]
        tunnel: w4 -> [w1872]
        stop <- w1873 stop-if-true
        # "Message loop"
        n234 = case shown="\"Receive\"" w1877 {
          tunnel: [w1883 w1903] -> w1871
          tunnel: [w1882 w1905] -> w1876
          tunnel: [w1890 w1900] -> w1875
          tunnel: w1874 -> [_ w1910]
          tunnel: w1872 -> [_ w1902]
          tunnel: [FALSE ("Stop RT Loops") w1901] -> w1873
          frame "Connect" {
            # "Attempts connection with the UI every 5 seconds, once successful, proceeds to Receive state."
            n235 = Bundle("", variant) -> (w1886:cluster{string, variant})  [unwired: 1 in]
            n236 = Create Network Stream Reader Endpoint(5:5000 ("timeout in ms (-1)"), 7:65536 ("reader buffer size"), 9:w1886, 11:"message reader" ("reader name")) -> (0:w1885:errorcluster, 3:w1881:refnum<k21>)  [unwired: 3 in]
            n237 = case shown="Error" w1885 {
              selector: w1885 -> [w1894 _]
              tunnel: [enum16{"Connect", "Receive"}."Receive" ("Message states") enum16{"Connect", "Receive"}."Connect" ("Message states")] -> w1890
              tunnel: [w1893 errorcluster {"status"=FALSE, "code"=0, "source"=""} ("error IO")] -> w1883
              tunnel: [w1895 refnum<k21> refnum ("reader name")] -> w1882
              tunnel: w1881 -> [w1895 _]
              frame No Error {
                n238 = shared-variable ".\\RT Variables.lvlib\\reader name"(w1895, error in=w1894) -> (error out=w1893:errorcluster)
              }
              frame Error {
              }
            }
          }
          frame "Receive" {
            # "Receives messages from the UI."
            n239 = shared-variable-read(w1910, w1902) -> (w1904:refnum<k21>, w1906:errorcluster, w1909:cluster{string, variant})  [unwired: 1 in, 1 out]
            n240 = Unbundle(w1909) -> (w1908:string, w1907:variant)
            n241 = case shown="\"HOME\"" w1908 {
              tunnel: w1907 -> [w1923 w1934 w1947 w1955 w1967 w1979 w1988 _]
              tunnel: w1906 -> [w1922 w1935 w1946 w1956 w1966 w1981 w1989 w1996]
              tunnel: [w1917 w1930 w1944 w1952 w1963 w1975 w1984 w1995] -> w1903
              tunnel: [w1921 w1936 w1950 w1960 w1971 refnum<k21> refnum ("reader name") w1992 refnum<k21> refnum ("reader name")] -> w1905
              tunnel: w1904 -> [w1921 w1936 w1950 w1960 w1971 w1974 w1992 w1994]
              tunnel: [FALSE ("Stop RT Loops") FALSE ("Stop RT Loops") FALSE ("Stop RT Loops") FALSE ("Stop RT Loops") FALSE ("Stop RT Loops") w1978 FALSE ("Stop RT Loops") FALSE ("Stop RT Loops")] -> w1901
              tunnel: [enum16{"Connect", "Receive"}."Receive" ("Message states") enum16{"Connect", "Receive"}."Receive" ("Message states") enum16{"Connect", "Receive"}."Receive" ("Message states") enum16{"Connect", "Receive"}."Receive" ("Message states") enum16{"Connect", "Receive"}."Receive" ("Message states") enum16{"Connect", "Receive"}."Receive" ("Message states") enum16{"Connect", "Receive"}."Receive" ("Message states") enum16{"Connect", "Receive"}."Connect" ("Message states")] -> w1900
              frame "GO1" {
                w1911 = TRUE
                w1915 = 0.0
                n242 = shared-variable ".\\RT Variables.lvlib\\RESET2V"(w1915) -> ()  [unwired: 1 in, 1 out]
                n243 = Variant To Data(error in=w1922, type=dbl[] [] ("appended array"), Variant=w1923) -> (data=w1913:dbl[], error out=w1918:errorcluster)
                n244 = Bundle("appended array"=w1913) -> (w1912:cluster{"appended array":dbl[]})  [unwired: 1 in]
                n245 = shared-variable ".\\RT Variables.lvlib\\RESET1V"(w1915) -> ()  [unwired: 1 in, 1 out]
                n246 = shared-variable ".\\RT Variables.lvlib\\D1"(w1912, error in=w1918) -> (error out=w1917:errorcluster)
                n247 = shared-variable ".\\RT Variables.lvlib\\HOMEV"(0.0) -> ()  [unwired: 1 in, 1 out]
                n248 = shared-variable ".\\RT Variables.lvlib\\Datos1_Recibidos"(w1911) -> ()  [unwired: 1 in, 1 out]
                n249 = shared-variable ".\\RT Variables.lvlib\\TCD_Indep"(w1911) -> ()  [unwired: 1 in, 1 out]
              }
              frame "GO2" {
                w1924 = TRUE
                w1928 = 0.0
                n250 = shared-variable ".\\RT Variables.lvlib\\RESET1V"(w1928) -> ()  [unwired: 1 in, 1 out]
                n251 = shared-variable ".\\RT Variables.lvlib\\RESET2V"(w1928) -> ()  [unwired: 1 in, 1 out]
                n252 = Variant To Data(error in=w1935, type=dbl[] [] ("appended array"), Variant=w1934) -> (data=w1927:dbl[], error out=w1931:errorcluster)
                n253 = Bundle("appended array"=w1927) -> (w1926:cluster{"appended array":dbl[]})  [unwired: 1 in]
                n254 = shared-variable ".\\RT Variables.lvlib\\D2"(w1926, error in=w1931) -> (error out=w1930:errorcluster)
                n255 = shared-variable ".\\RT Variables.lvlib\\HOMEV"(0.0) -> ()  [unwired: 1 in, 1 out]
                n256 = shared-variable ".\\RT Variables.lvlib\\TCD_Indep"(w1924) -> ()  [unwired: 1 in, 1 out]
                n257 = shared-variable ".\\RT Variables.lvlib\\Datos2_Recibidos"(w1924) -> ()  [unwired: 1 in, 1 out]
              }
              frame "GO3" {
                w1942 = 0.0
                n258 = shared-variable ".\\RT Variables.lvlib\\RESET2V"(w1942) -> ()  [unwired: 1 in, 1 out]
                n259 = Variant To Data(error in=w1946, type=dbl[] [] ("appended array"), Variant=w1947) -> (data=w1939:dbl[], error out=w1945:errorcluster)
                n260 = Bundle("appended array"=w1939) -> (w1938:cluster{"appended array":dbl[]})  [unwired: 1 in]
                n261 = shared-variable ".\\RT Variables.lvlib\\D1"(w1938, error in=w1945) -> (error out=w1944:errorcluster)
                n262 = shared-variable ".\\RT Variables.lvlib\\RESET1V"(w1942) -> ()  [unwired: 1 in, 1 out]
                n263 = shared-variable ".\\RT Variables.lvlib\\HOMEV"(0.0) -> ()  [unwired: 1 in, 1 out]
                n264 = shared-variable ".\\RT Variables.lvlib\\TCD_Indep"(FALSE) -> ()  [unwired: 1 in, 1 out]
                n265 = shared-variable ".\\RT Variables.lvlib\\Datos1_Recibidos"(TRUE) -> ()  [unwired: 1 in, 1 out]
              }
              frame "HOME" {
                w1951 = 0.0
                n266 = Variant To Data(error in=w1956, type=0.0, Variant=w1955) -> (data=w1954:dbl, error out=w1953:errorcluster)
                n267 = shared-variable ".\\RT Variables.lvlib\\RESET2V"(w1951) -> ()  [unwired: 1 in, 1 out]
                n268 = shared-variable ".\\RT Variables.lvlib\\HOMEV"(w1954, error in=w1953) -> (error out=w1952:errorcluster)
                n269 = shared-variable ".\\RT Variables.lvlib\\RESET1V"(w1951) -> ()  [unwired: 1 in, 1 out]
              }
              frame "RESET2" {
                n270 = shared-variable ".\\RT Variables.lvlib\\RESET1V"(0.0) -> ()  [unwired: 1 in, 1 out]
                n271 = Variant To Data(error in=w1966, type=0.0, Variant=w1967) -> (data=w1964:dbl, error out=w1965:errorcluster)
                n272 = shared-variable ".\\RT Variables.lvlib\\RESET2V"(w1964, error in=w1965) -> (error out=w1963:errorcluster)
                n273 = shared-variable ".\\RT Variables.lvlib\\HOMEV"(0.0) -> ()  [unwired: 1 in, 1 out]
              }
              frame "Stop" {
                n274 = Variant To Data(error in=w1981, type=TRUE ("Stop RT Loops"), Variant=w1979) -> (data=w1978:bool, error out=w1980:errorcluster)
                n275 = shared-variable ".\\RT Variables.lvlib\\Stop RT Loops"(w1978, error in=w1980) -> (error out=w1976:errorcluster)
                n276 = Destroy Stream Endpoint(8:w1976, 11:w1974) -> (0:w1975:errorcluster)
              }
              frame "RESET1" {
                n277 = shared-variable ".\\RT Variables.lvlib\\RESET2V"(0.0) -> ()  [unwired: 1 in, 1 out]
                n278 = Variant To Data(error in=w1989, type=0.0, Variant=w1988) -> (data=w1986:dbl, error out=w1985:errorcluster)
                n279 = shared-variable ".\\RT Variables.lvlib\\RESET1V"(w1986, error in=w1985) -> (error out=w1984:errorcluster)
                n280 = shared-variable ".\\RT Variables.lvlib\\HOMEV"(0.0) -> ()  [unwired: 1 in, 1 out]
              }
              frame "Disconnect UI", Default {
                n281 = Destroy Stream Endpoint(8:w1996, 11:w1994) -> (0:w1995:errorcluster)
              }
            }
          }
        }
        n282 = case shown="Error" w1871 {
          selector: w1871 -> [w1878 w1879]
          tunnel: [w1878 w1879] -> w1870
          frame No Error {
            # "No action required."
          }
          frame Error {
            # "Stops RT in case of error."
            n283 = shared-variable ".\\RT Variables.lvlib\\Stop RT Loops"(TRUE ("Stop RT Loops")) -> ()  [unwired: 1 in, 1 out]
          }
        }
      }
      n284 = while {
        shift-right: [w1825] -> w42
        shift-left: refnum<k21> refnum ("writer endpoint") -> [w1823]
        tunnel: [w1824] -> w43
        tunnel: w4 -> [w1822]
        shift-right: [w1821] -> _
        shift-left: enum16{"Connect", "Send"}."Connect" ("Message states") -> [w1826]
        stop <- w1827 stop-if-true
        # "Data sending loop"
        n285 = case shown="\"Send\"" w1826 {
          tunnel: [w1830 w1846] -> w1824
          tunnel: [w1828 w1844] -> w1825
          tunnel: [w1835 w1847] -> w1821
          tunnel: w1823 -> [_ w1853]
          tunnel: w1822 -> [w1831 w1852]
          frame "Connect" {
            # "Attempts connection with the UI every 5 seconds, once successful, proceeds to Send state."
            n286 = Create Network Stream Writer Endpoint(5:5000 ("timeout in ms (-1)"), 7:4096 ("writer buffer size"), 8:w1831, 9:T6 {"Double"=0.0, "dbl Scaled Value"=0.0, "Output"=0.0, "seconds since 1Jan1904"=timestamp(0 s since 1904-01-01)} ("Data"), 11:"data writer" ("writer name")) -> (0:w1833:errorcluster, 3:w1829:refnum<k21>)  [unwired: 2 in]
            n287 = case shown="No Error" w1833 {
              selector: w1833 -> [w1838 _]
              tunnel: [enum16{"Connect", "Send"}."Send" ("Message states") enum16{"Connect", "Send"}."Connect" ("Message states")] -> w1835
              tunnel: [w1838 errorcluster {"status"=FALSE, "code"=0, "source"=""} ("error IO")] -> w1830
              tunnel: w1829 -> [w1840 _]
              tunnel: [w1840 refnum<k21> refnum ("writer endpoint")] -> w1828
              frame No Error {
              }
              frame Error {
              }
            }
          }
          frame "Send" {
            # "Sends deterministic loop acquired data to the UI."
            n288 = shared-variable ".\\RT Variables.lvlib\\Data"(error in=w1852) -> (w1849:T6, error out=w1851:errorcluster)
            n289 = Unbundle By Name(w1851) -> ("code"=w1850:i32)
            n290 = case shown="0, Default" w1850 {
              tunnel: [w1866 w1868] -> w1848
              tunnel: [w1865 w1867] -> w1845
              tunnel: w1853 -> [w1864 w1867]
              tunnel: w1851 -> [w1863 w1868]
              tunnel: w1849 -> [w1862 _]
              frame 0, Default {
                n291 = shared-variable-write(w1864, w1863, w1862) -> (w1865:refnum<k21>, w1866:errorcluster)  [unwired: 1 in, 1 out]
              }
              frame -2220 {
                n292 = Wait (ms)(milliseconds to wait=u32 10) -> ()  [unwired: 1 out]
              }
            }
            n293 = case shown="No Error" w1848 {
              selector: w1848 -> [w1856 w1860]
              tunnel: [enum16{"Connect", "Send"}."Send" ("Message states") enum16{"Connect", "Send"}."Connect" ("Message states")] -> w1847
              tunnel: [w1856 errorcluster {"status"=FALSE, "code"=0, "source"=""} ("error IO")] -> w1846
              tunnel: w1845 -> [w1854 w1859]
              tunnel: [w1854 refnum<k21> refnum ("writer endpoint")] -> w1844
              frame No Error {
              }
              frame Error {
                n294 = Destroy Stream Endpoint(8:w1860, 11:w1859) -> ()  [unwired: 1 out]
              }
            }
          }
        }
        n295 = shared-variable ".\\RT Variables.lvlib\\Stop RT Loops"() -> (w1827:bool)  [unwired: 1 in, 1 out]
      }
      n296 = Destroy Stream Endpoint(8:w43, 11:w42) -> (0:w40:errorcluster)
      n297 = node-c288(w48) -> ()  [unwired: 1 out]
      n298 = case shown="Error" w7 {
        selector: w7 -> [w1818 w1819]
        tunnel: [w1818 w1819] -> w35
        frame No Error {
          # "No action required."
        }
        frame Error {
          # "Destroys Message network stream to stop Message loop, in case of error."
          n299 = shared-variable ".\\RT Variables.lvlib\\reader name"() -> (w1820:refnum<k21>)  [unwired: 1 in, 1 out]
          n300 = Destroy Stream Endpoint(11:w1820) -> ()  [unwired: 1 in, 1 out]
        }
      }
      n301 = Merge Errors(w40, w39, w35, w6, w5) -> (w38:errorcluster)
      n302 = shared-variable "myRIO-1900\\Network Shared Variables.lvlib\\error IO"(w38) -> ()  [unwired: 1 in, 1 out]
      "Tiempo de muestreo" <- 0.005 ("Tiempo de muestreo")
      "Kp1" <- 0.0036 ("Kp1")
      "Ti1" <- 0.471 ("Ti")
      "Td1" <- 0.119 ("Td")
      "Kp2" <- 0.0022 ("Kp1")
      "Ti2" <- 0.471 ("Ti")
      "Td2" <- 0.1184 ("Td")
    }
    frame #1 {
      n303 = call <vilib>:"Reset myRIO.vi"() -> ()  [unwired: 11 in, 1 out]
    }
  }
